vi "read_back.vi"() -> ()   [LabVIEW 2021]
panel:
  in  "stop":bool
  in  "Set Settings":bool
  in  "VISA resource name":refnum<visa-resource-name>
  in  "CH2":T1={"Scale"=1.0, "Position"=0.0, "Toggle"=FALSE}
  in  "CH1":T1={"Scale"=1.0, "Position"=0.0, "Toggle"=FALSE}
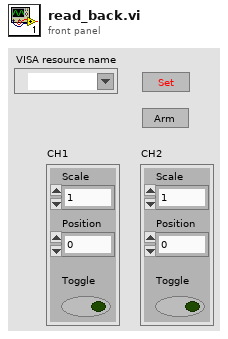
[diagram p1: front panel]
types:
  T1 = cluster{"Scale":dbl, "Position":dbl, "Toggle":bool}
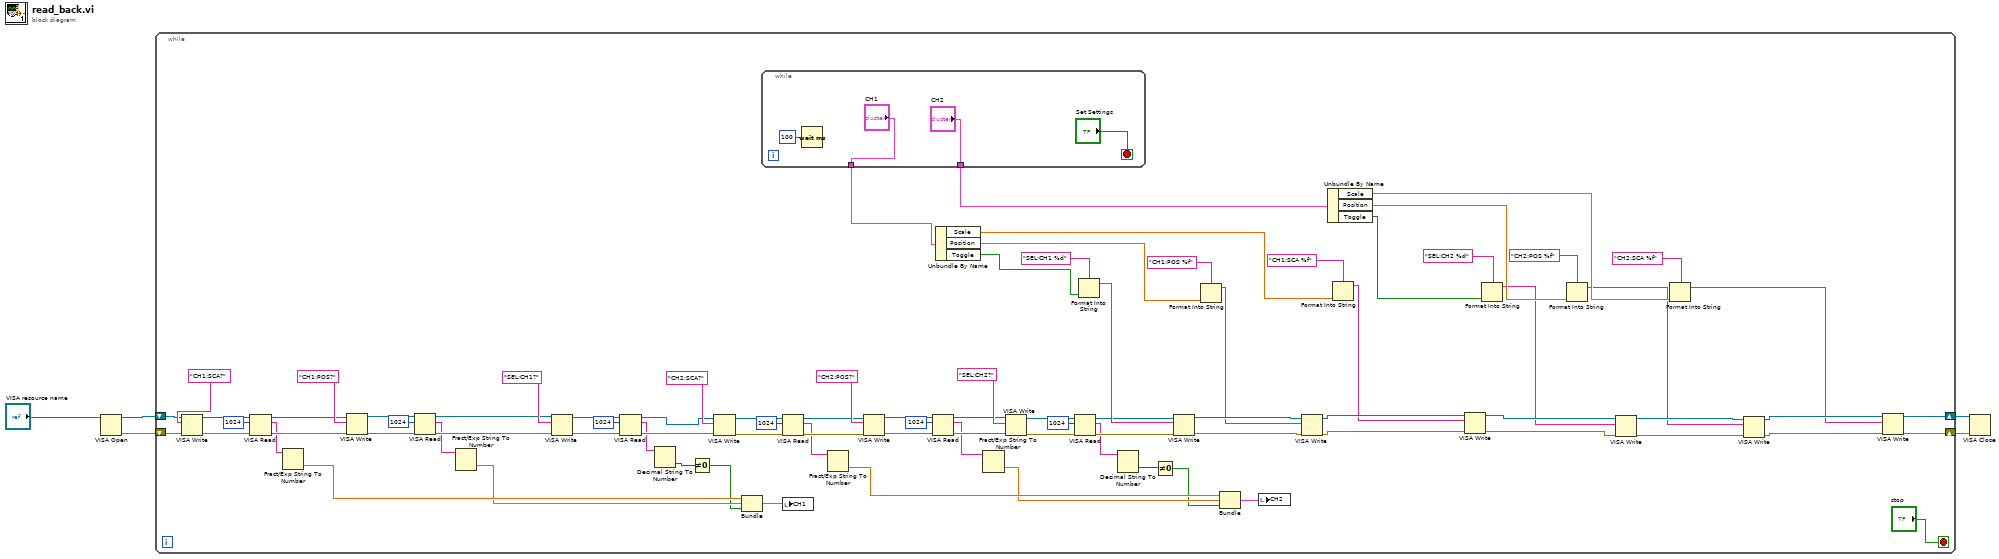
[diagram p0: block diagram]
diagram:
  n1 = VISA Open(VISA resource name="VISA resource name") -> (VISA resource name=w2:refnum<visa-resource-name>, error out=w1:errorcluster)  [unwired: 4 in]
  n2 = while {
    shift-right: [w82] -> w4
    shift-left: w2 -> [w58]
    shift-right: [w6] -> w3
    shift-left: w1 -> [w57]
    stop <- "stop" stop-if-true
    n3 = VISA Write(VISA resource name=w58, write buffer="CH1:SCA?", error in (no error)=w57) -> (VISA resource name out=w61:refnum<visa-resource-name>, error out=w60:errorcluster)  [unwired: 1 out]
    n4 = VISA Read(VISA resource name=w61, byte count=u32 1024, error in (no error)=w60) -> (VISA resource name out=w35:refnum<visa-resource-name>, read buffer=w23:string, error out=w34:errorcluster)  [unwired: 1 out]
    n5 = Fract/Exp String To Number(string=w23) -> (number=w15:dbl)  [unwired: 3 in, 1 out]
    n6 = VISA Write(VISA resource name=w35, write buffer="CH1:POS?", error in (no error)=w34) -> (VISA resource name out=w48:refnum<visa-resource-name>, error out=w47:errorcluster)  [unwired: 1 out]
    n7 = VISA Read(VISA resource name=w48, byte count=u32 1024, error in (no error)=w47) -> (VISA resource name out=w33:refnum<visa-resource-name>, read buffer=w22:string, error out=w32:errorcluster)  [unwired: 1 out]
    n8 = Fract/Exp String To Number(string=w22) -> (number=w14:dbl)  [unwired: 3 in, 1 out]
    n9 = VISA Write(VISA resource name=w33, write buffer="SEL:CH1?", error in (no error)=w32) -> (VISA resource name out=w54:refnum<visa-resource-name>, error out=w53:errorcluster)  [unwired: 1 out]
    n10 = VISA Read(VISA resource name=w54, byte count=u32 1024, error in (no error)=w53) -> (VISA resource name out=w31:refnum<visa-resource-name>, read buffer=w21:string, error out=w30:errorcluster)  [unwired: 1 out]
    n11 = Decimal String To Number(string=w21) -> (number=w17:i32)  [unwired: 2 in, 1 out]
    n12 = Not Equal To 0?(x=w17) -> (x != 0?=w13:bool)
    n13 = VISA Write(VISA resource name=w31, write buffer="CH2:SCA?", error in (no error)=w30) -> (VISA resource name out=w52:refnum<visa-resource-name>, error out=w51:errorcluster)  [unwired: 1 out]
    n14 = Bundle(w15, w14, w13) -> (w12:cluster{dbl, dbl, bool})  [unwired: 1 in]
    n15 = while {
      tunnel: ["CH2"] -> w63
      tunnel: ["CH1"] -> w59
      stop <- "Set Settings" stop-if-true
      n16 = Wait (ms)(milliseconds to wait=u32 100) -> ()  [unwired: 1 out]
    }
    n17 = local write "CH1"(w12) -> ()
    n18 = VISA Read(VISA resource name=w52, byte count=u32 1024, error in (no error)=w51) -> (VISA resource name out=w29:refnum<visa-resource-name>, read buffer=w20:string, error out=w28:errorcluster)  [unwired: 1 out]
    n19 = Fract/Exp String To Number(string=w20) -> (number=w11:dbl)  [unwired: 3 in, 1 out]
    n20 = VISA Write(VISA resource name=w29, write buffer="CH2:POS?", error in (no error)=w28) -> (VISA resource name out=w50:refnum<visa-resource-name>, error out=w49:errorcluster)  [unwired: 1 out]
    n21 = VISA Read(VISA resource name=w50, byte count=u32 1024, error in (no error)=w49) -> (VISA resource name out=w27:refnum<visa-resource-name>, read buffer=w19:string, error out=w26:errorcluster)  [unwired: 1 out]
    n22 = Unbundle By Name(w59) -> ("Scale"=w73:dbl, "Position"=w74:dbl, "Toggle"=w75:bool)
    n23 = Fract/Exp String To Number(string=w19) -> (number=w10:dbl)  [unwired: 3 in, 1 out]
    n24 = VISA Write(VISA resource name=w27, write buffer="SEL:CH2?", error in (no error)=w26) -> (VISA resource name out=w56:refnum<visa-resource-name>, error out=w55:errorcluster)  [unwired: 1 out]
    n25 = VISA Read(VISA resource name=w56, byte count=u32 1024, error in (no error)=w55) -> (VISA resource name out=w25:refnum<visa-resource-name>, read buffer=w18:string, error out=w24:errorcluster)  [unwired: 1 out]
    n26 = Format Into String(format string="SEL:CH1 %d", w75) -> (resulting string=w69:string)  [unwired: 2 in, 1 out]
    n27 = Decimal String To Number(string=w18) -> (number=w16:i32)  [unwired: 2 in, 1 out]
    n28 = Not Equal To 0?(x=w16) -> (x != 0?=w9:bool)
    n29 = VISA Write(VISA resource name=w25, write buffer=w69, error in (no error)=w24) -> (VISA resource name out=w89:refnum<visa-resource-name>, error out=w90:errorcluster)  [unwired: 1 out]
    n30 = Format Into String(format string="CH1:POS %f", w74) -> (resulting string=w68:string)  [unwired: 2 in, 1 out]
    n31 = Bundle(w11, w10, w9) -> (w8:cluster{dbl, dbl, bool})  [unwired: 1 in]
    n32 = local write "CH2"(w8) -> ()
    n33 = VISA Write(VISA resource name=w89, write buffer=w68, error in (no error)=w90) -> (VISA resource name out=w91:refnum<visa-resource-name>, error out=w92:errorcluster)  [unwired: 1 out]
    n34 = Unbundle By Name(w63) -> ("Scale"=w70:dbl, "Position"=w71:dbl, "Toggle"=w72:bool)
    n35 = Format Into String(format string="CH1:SCA %f", w73) -> (resulting string=w67:string)  [unwired: 2 in, 1 out]
    n36 = VISA Write(VISA resource name=w91, write buffer=w67, error in (no error)=w92) -> (VISA resource name out=w84:refnum<visa-resource-name>, error out=w83:errorcluster)  [unwired: 1 out]
    n37 = Format Into String(format string="SEL:CH2 %d", w72) -> (resulting string=w66:string)  [unwired: 2 in, 1 out]
    n38 = Format Into String(format string="CH2:POS %f", w71) -> (resulting string=w65:string)  [unwired: 2 in, 1 out]
    n39 = VISA Write(VISA resource name=w84, write buffer=w66, error in (no error)=w83) -> (VISA resource name out=w85:refnum<visa-resource-name>, error out=w86:errorcluster)  [unwired: 1 out]
    n40 = Format Into String(format string="CH2:SCA %f", w70) -> (resulting string=w64:string)  [unwired: 2 in, 1 out]
    n41 = VISA Write(VISA resource name=w85, write buffer=w65, error in (no error)=w86) -> (VISA resource name out=w87:refnum<visa-resource-name>, error out=w88:errorcluster)  [unwired: 1 out]
    n42 = VISA Write(VISA resource name=w87, write buffer=w64, error in (no error)=w88) -> (VISA resource name out=w82:refnum<visa-resource-name>, error out=w6:errorcluster)  [unwired: 1 out]
  }
  n43 = VISA Close(VISA resource name=w4, error in (no error)=w3) -> ()  [unwired: 1 out]
